vi "Main.vi"() -> ()   [LabVIEW 2015]
uses:
  TypeDefs/Buttons UI.ctl
  TypeDefs/States.ctl
  TypeDefs/Acq Loop Data.ctl
panel:
  in  "#samples":dbl=100.0
  in  "Frequency":dbl=1000.0
  out "File Path":path
  in  "File Name Prefix":string="LV Academy"
  in  "Buttons":T1
  out "Wykres":dbl[](graph)
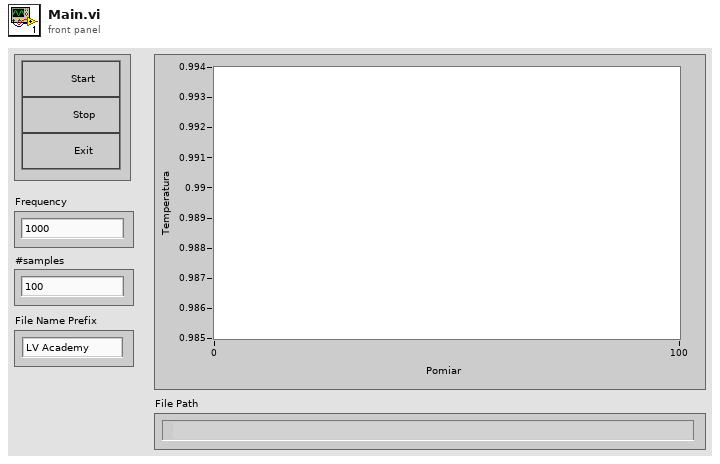
[diagram p1: front panel]
types:
  T1 = typedef "Buttons UI.ctl" = cluster{"Start":bool, "Stop":bool, "Exit":bool}
  T2 = typedef "Acq Loop Data.ctl" = cluster{"File Name Profix":string, "Frequency":dbl, "#samples":i32, "DAQ task ":refnum<k21>}
  T3 = typedef "Queue Data" = cluster{"Action":string, "Data":dbl[]}
  T4 = typedef "States.ctl" = enum16{"Check if Stop or Exit", "Exit", "Wait for Start or Exit", "Start Acquisition", "Reset Acquisition", "Acquisition"}
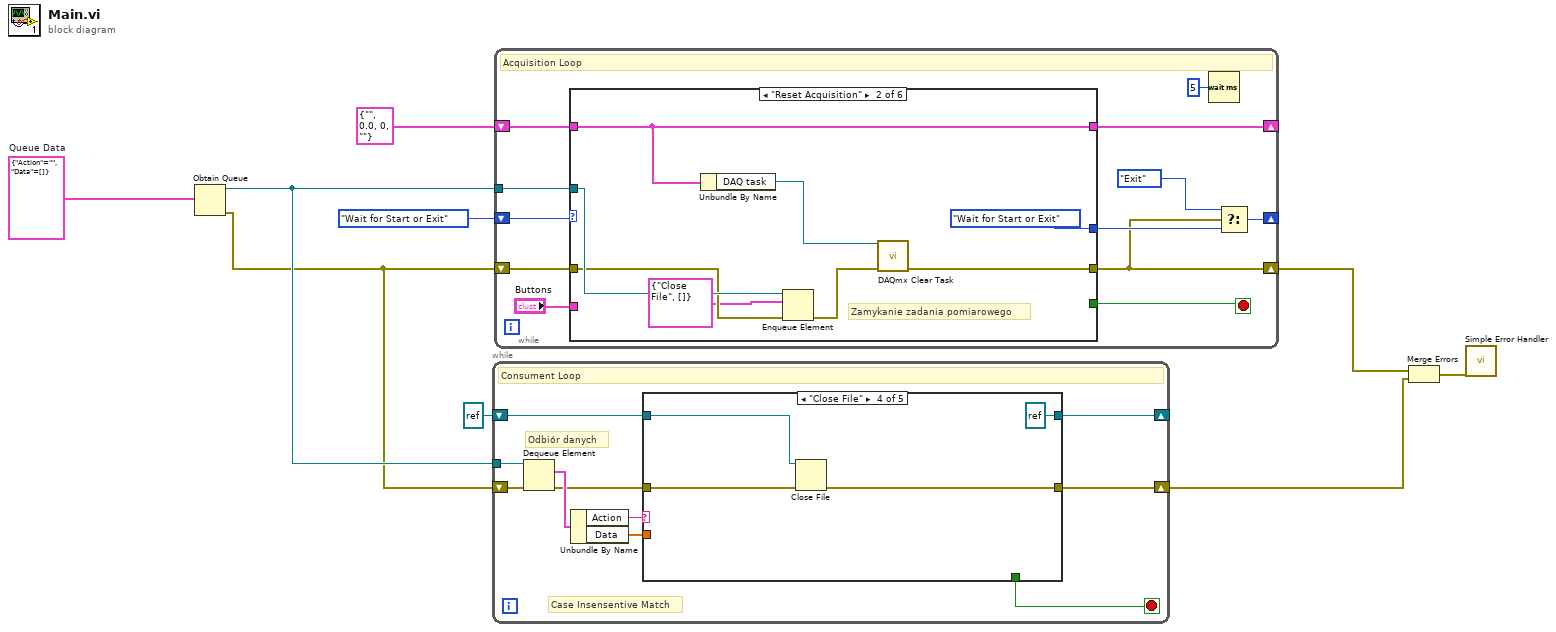
[diagram p0: block diagram]
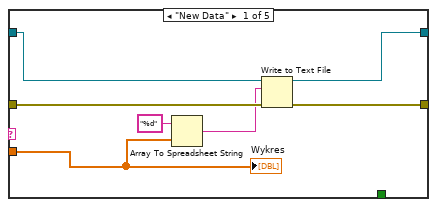
[diagram p2: hidden frame]
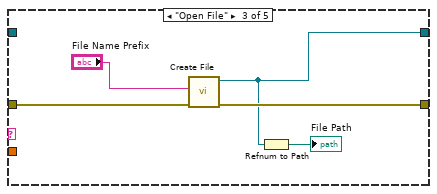
[diagram p4: hidden frame]
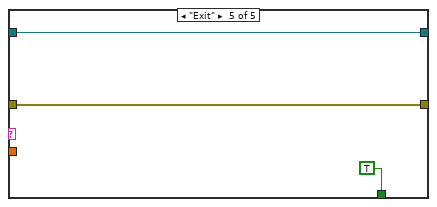
[diagram p5: hidden frame]
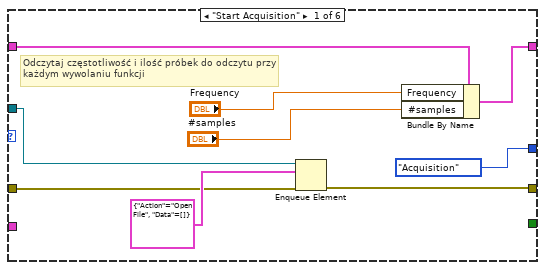
[diagram p6: hidden frame]
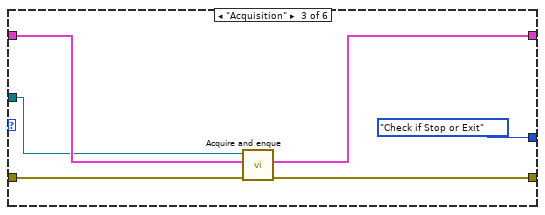
[diagram p7: hidden frame]
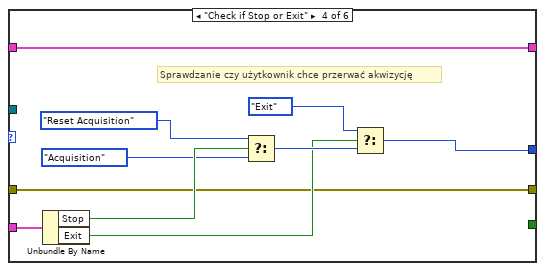
[diagram p8: hidden frame]
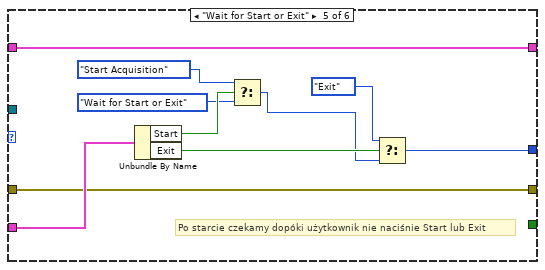
[diagram p9: hidden frame]
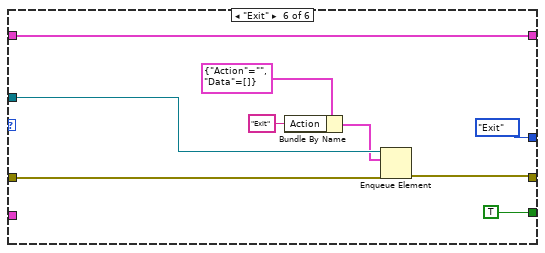
[diagram p10: hidden frame]
diagram:
  w3 = T3 {"Action"="", "Data"=[]}  # Queue Data
  n1 = Obtain Queue(element data type=w3) -> (queue out=w2:refnum<queue>, error out=w1:errorcluster)  [unwired: 4 in, 1 out]
  n2 = while {
    shift-right: [w13] -> w6
    shift-left: w1 -> [w19]
    shift-right: [w14] -> _
    shift-left: refnum<file> refnum ("refnum out") -> [w12]
    tunnel: w2 -> [w10]
    stop <- w11 stop-if-true
    # "Odbiór danych"
    # "Case Insensentive Match"
    # "Consument Loop"
    n3 = Dequeue Element(queue=w10, error in (no error)=w19) -> (element=w18:T3, error out=w15:errorcluster)  [unwired: 1 in, 2 out]
    n4 = Unbundle By Name(w18) -> ("Action"=w17:string, "Data"=w16:dbl[])
    n5 = case shown="\"Close File\"" w17 {
      tunnel: w16 -> [w22 _ _ _ _]
      tunnel: w15 -> [w26 w28 w33 w37 w39]
      tunnel: [w23 w27 w29 refnum<file> refnum ("refnum out") w38] -> w14
      tunnel: [w25 w28 w31 w35 w39] -> w13
      tunnel: w12 -> [w24 w27 _ w36 w38]
      tunnel: [_ _ _ _ TRUE] -> w11
      frame "New Data" {
        n6 = Array To Spreadsheet String(array=w22, 3:"%d" ("format string")) -> (spreadsheet string=w21:string)  [unwired: 1 in]
        n7 = Write to Text File(file (use dialog)=w24, text=w21, error in=w26) -> (refnum out=w23:refnum<file>, error out=w25:errorcluster)  [unwired: 1 in, 1 out]
        "Wykres" <- w22
      }
      frame Default {
      }
      frame "Open File" {
        n8 = call "Create File.vi"("error in (no error)"=w33, "File Name Prefix"="File Name Prefix") -> ("error out"=w31:errorcluster, "refnum out"=w29:refnum<file>)  [unwired: 8 in]
        n9 = Refnum to Path(1:w29) -> (0:→"File Path":path)
      }
      frame "Close File" {
        n10 = Close File(refnum=w36, error in=w37) -> (error out=w35:errorcluster)  [unwired: 1 out]
      }
      frame "Exit" {
      }
    }
  }
  n11 = while {
    shift-right: [w44] -> _
    shift-left: States."Wait for Start or Exit" -> [w52]
    shift-right: [w48] -> _
    shift-left: T2 {"File Name Profix"="", "Frequency"=0.0, "#samples"=0, "DAQ task "=""} -> [w49]
    shift-right: [w42] -> w5
    shift-left: w1 -> [w51]
    tunnel: w2 -> [w41]
    stop <- w46 stop-if-true
    # "Acquisition Loop"
    n12 = case shown="\"Reset Acquisition\"" w52 {
      tunnel: w51 -> [w54 w64 w75 w77 w88 w97]
      tunnel: "Buttons" -> [_ _ _ w85 w95 _]
      tunnel: [States."Acquisition" States."Wait for Start or Exit" States."Check if Stop or Exit" w78 w90 States."Exit"] -> w45
      tunnel: w49 -> [w61 w66 w74 w76 w89 w101]
      tunnel: [w58 w66 w71 w76 w89 w101] -> w48
      tunnel: [w53 w69 w73 w77 w88 w96] -> w42
      tunnel: [_ _ _ _ _ TRUE] -> w46
      tunnel: w41 -> [w56 w65 w70 _ _ w99]
      frame "Start Acquisition" {
        # "Odczytaj częstotliwość i ilość próbek do odczytu przy każdym wywolaniu funkcji"
        n13 = Enqueue Element(queue=w56, element=T3 {"Action"="Open File", "Data"=[]}, error in (no error)=w54) -> (error out=w53:errorcluster)  [unwired: 1 in, 2 out]
        n14 = Bundle By Name(cluster=w61, "Frequency"="Frequency", "#samples"="#samples") -> (w58:T2)
      }
      frame "Reset Acquisition" {
        # "Zamykanie zadania pomiarowego"
        n15 = Unbundle By Name(w66) -> ("DAQ task"=w68:refnum<k21>)
        n16 = Enqueue Element(queue=w65, element=T3 {"Action"="Close File", "Data"=[]}, error in (no error)=w64) -> (error out=w62:errorcluster)  [unwired: 1 in, 2 out]
        n17 = call <vilib>:"DAQmx Clear Task.vi"("task in"=w68, "error in"=w62) -> ("error out"=w69:errorcluster)  [unwired: 13 in]
      }
      frame "Acquisition" {
        n18 = call "Acquire and enque.vi"("error in (no error)"=w75, "Data In"=w74, "Queue in"=w70) -> ("error out"=w73:errorcluster, "Data Out"=w71:T2)  [unwired: 7 in]
      }
      frame "Check if Stop or Exit" {
        # "Sprawdzanie czy użytkownik chce przerwać akwizycję"
        n19 = Unbundle By Name(w85) -> ("Stop"=w84:bool, "Exit"=w80:bool)
        n20 = Select(t=States."Reset Acquisition", s=w84, f=States."Acquisition") -> (s? t:f=w81:T4)
        n21 = Select(t=States."Exit", s=w80, f=w81) -> (s? t:f=w78:T4)
      }
      frame "Wait for Start or Exit" {
        # "Po starcie czekamy dopóki użytkownik nie naciśnie Start lub Exit"
        n22 = Unbundle By Name(w95) -> ("Start"=w94:bool, "Exit"=w91:bool)
        n23 = Select(t=States."Start Acquisition", s=w94, f=States."Wait for Start or Exit") -> (s? t:f=w87:T4)
        n24 = Select(t=States."Exit", s=w91, f=w87) -> (s? t:f=w90:T4)
      }
      frame "Exit" {
        n25 = Bundle By Name(cluster=T3 {"Action"="", "Data"=[]}, "Action"="Exit") -> (w98:T3)
        n26 = Enqueue Element(queue=w99, element=w98, error in (no error)=w97) -> (error out=w96:errorcluster)  [unwired: 1 in, 2 out]
      }
    }
    n27 = Wait (ms)(milliseconds to wait=u32 5) -> ()  [unwired: 1 out]
    n28 = Select(t=States."Exit", s=w42, f=w45) -> (s? t:f=w44:T4)
  }
  n29 = Merge Errors(w5, w6) -> (w4:errorcluster)
  n30 = call <vilib>:"Simple Error Handler.vi"("error in (no error)"=w4) -> ()  [unwired: 4 in, 5 out]
